vi "主界面.vi"() -> ()   [LabVIEW 2018]
panel:
  in  "配置文件":path=path "D:/Labviewprogram/多账户登录"
  in  "修改密码":bool
  in  "进入系统":bool
  in  "用户管理":bool
  in  "退出":bool
  in  "登录":bool
  in  "密 码":string
  in  "账 户":u16(ring)
  # "登录系统"
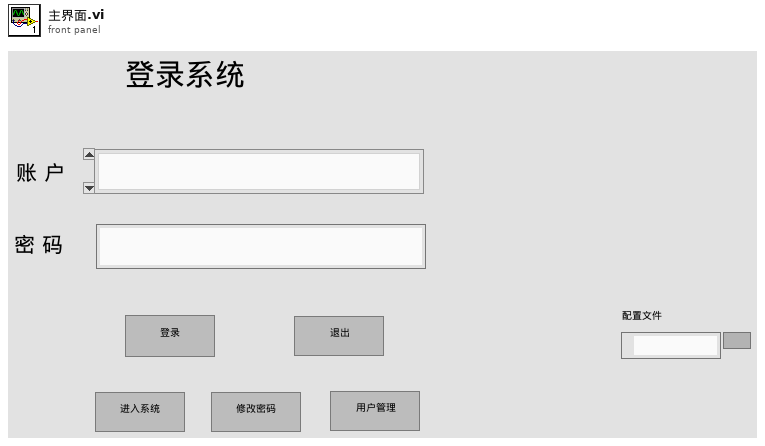
[diagram p1: front panel]
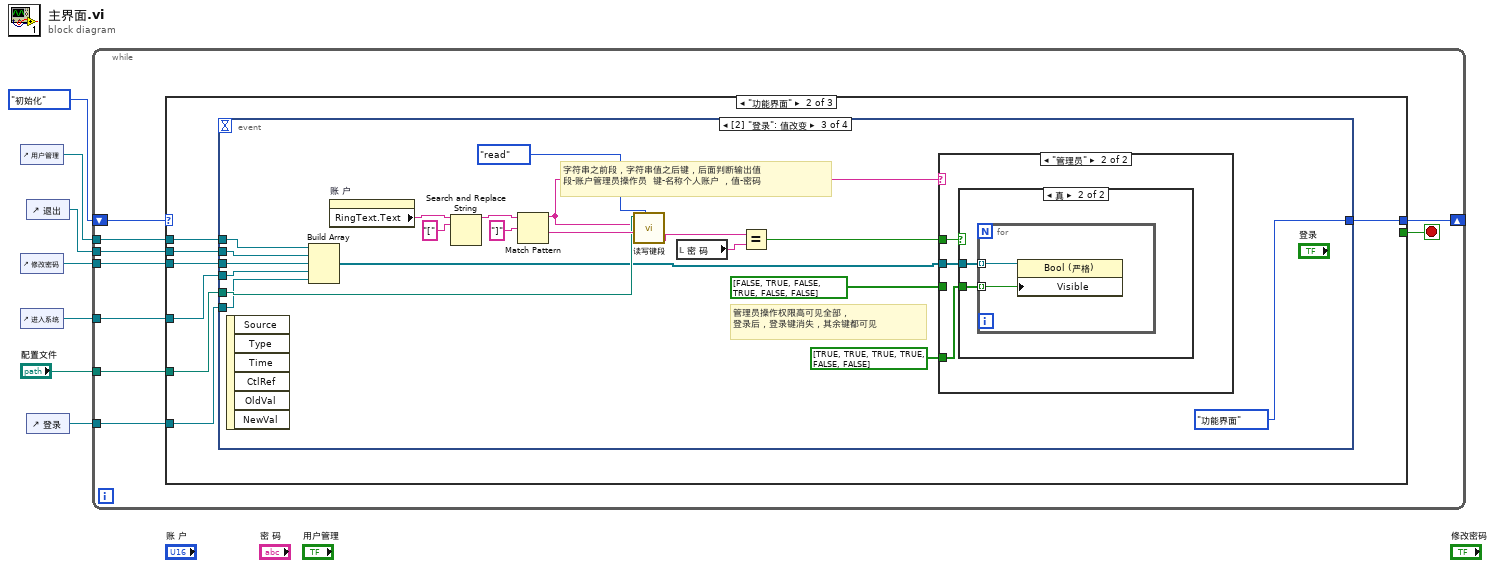
[diagram p0: block diagram]
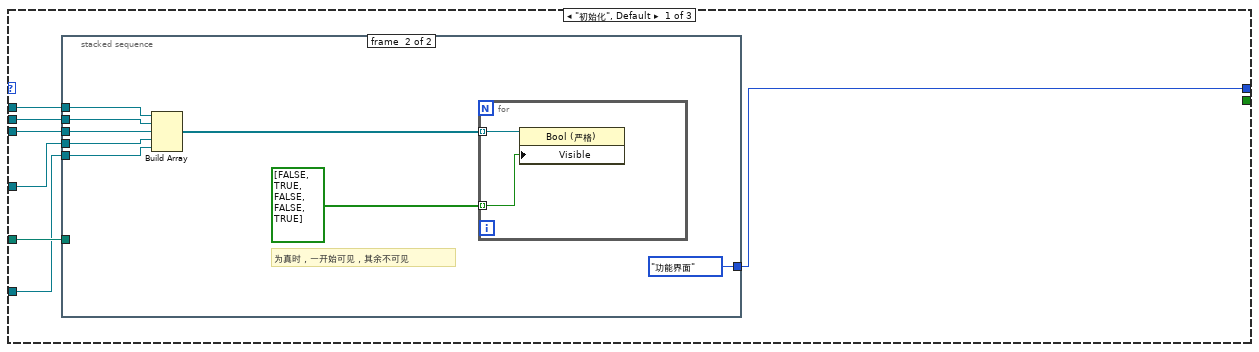
[diagram p2: hidden frame]
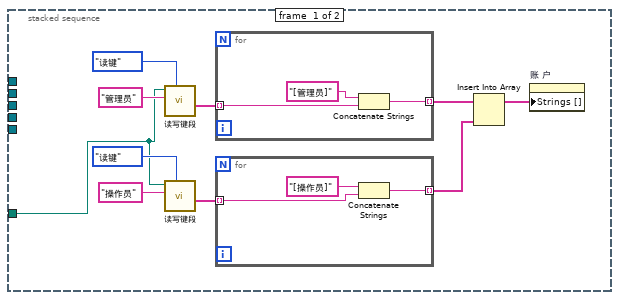
[diagram p3: hidden frame]
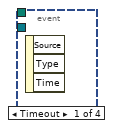
[diagram p4: hidden frame]
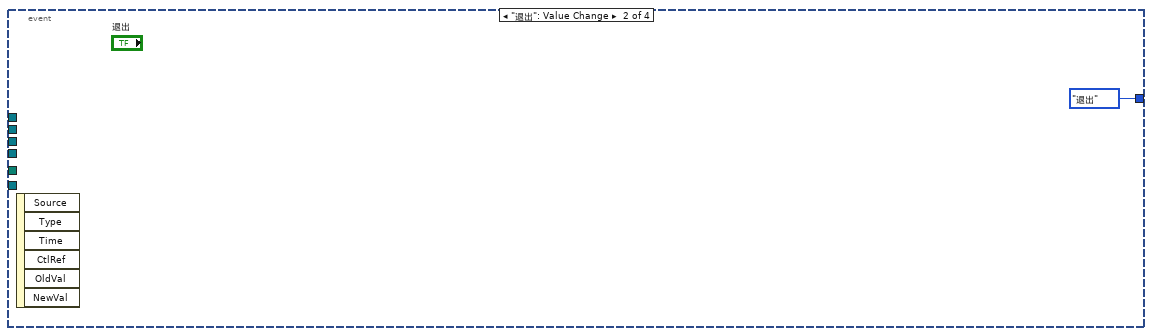
[diagram p5: hidden frame]
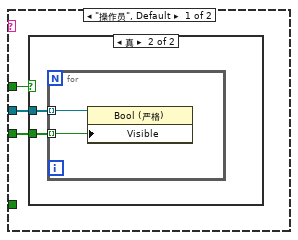
[diagram p6: hidden frame]
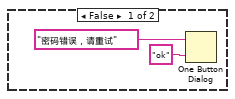
[diagram p7: hidden frame]
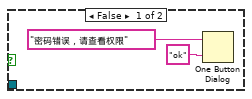
[diagram p8: hidden frame]
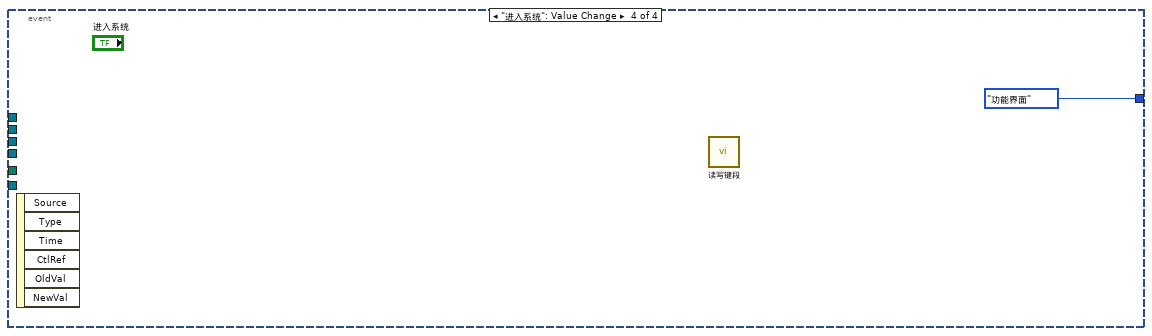
[diagram p9: hidden frame]
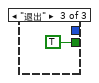
[diagram p10: hidden frame]
diagram:
  n1 = control-ref of="用户管理"() -> (w5:refnum<vi>)
  n2 = control-ref of="修改密码"() -> (w3:refnum<vi>)
  n3 = control-ref of="进入系统"() -> (w2:refnum<vi>)
  n4 = control-ref of="退出"() -> (w4:refnum<vi>)
  n5 = control-ref of="登录"() -> (w1:refnum<vi>)
  n6 = while {
    shift-right: [w9] -> _
    shift-left: enum16{"初始化", "功能界面", "退出"}."初始化" ("枚举") -> [w16]
    tunnel: "配置文件" -> [w15]
    tunnel: w5 -> [w14]
    tunnel: w4 -> [w13]
    tunnel: w3 -> [w12]
    tunnel: w2 -> [w11]
    tunnel: w1 -> [w10]
    stop <- w8 stop-if-true
    n7 = case shown="\"功能界面\"" w16 {
      tunnel: w15 -> [w23 w55 _]
      tunnel: w14 -> [w22 w54 _]
      tunnel: w13 -> [w21 w53 _]
      tunnel: w12 -> [w20 w52 _]
      tunnel: w11 -> [w19 w51 _]
      tunnel: w10 -> [w18 w50 _]
      tunnel: [w17 w56 _] -> w9
      tunnel: [_ _ TRUE] -> w8
      frame "初始化", Default {
        n8 = stacked-sequence {
          tunnel: w23 -> [w27 _]
          tunnel: w22 -> [_ w47]
          tunnel: w21 -> [_ w46]
          tunnel: w20 -> [_ w45]
          tunnel: w19 -> [_ w44]
          tunnel: w18 -> [_ w43]
          tunnel: [_ enum16{"初始化", "功能界面", "退出"}."功能界面" ("枚举")] -> w17
          frame #0 {
            n9 = call "读写键段.vi"("枚举"=enum16{"write", "read", "读键", "读段"}."读键", "段"="管理员", "配置文件"=w27) -> ("键名"=w31:string[])  [unwired: 6 in, 2 out]
            n10 = call "读写键段.vi"("枚举"=enum16{"write", "read", "读键", "读段"}."读键", "段"="操作员", "配置文件"=w27) -> ("键名"=w30:string[])  [unwired: 6 in, 2 out]
            n11 = for {
              tunnel: w31 -> [w38] mode=indexing
              tunnel: [w37] -> w26 mode=indexing
              n12 = Concatenate Strings("[管理员]" ("字符串"), w38) -> (w37:string)
            }
            n13 = for {
              tunnel: w30 -> [w35] mode=indexing
              tunnel: [w34] -> w25 mode=indexing
              n14 = Concatenate Strings("[操作员]" ("字符串"), w35) -> (w34:string)
            }
            n15 = Insert Into Array(array=w26, new element=w25) -> (w24:string[])  [unwired: 1 in]
            n16 = property on="账 户" class="Ring (严格)"("Strings []"=w24) -> ()  [unwired: 2 in, 2 out]
          }
          frame #1 {
            # "为真时，一开始可见，其余不可见"
            n17 = Build Array(w47, w46, w45, w44, w43) -> (w42:refnum<vi>[])
            n18 = for {
              tunnel: w42 -> [w49] mode=indexing
              tunnel: bool[] [FALSE, TRUE, FALSE, FALSE, TRUE] -> [w48] mode=indexing
              n19 = property class="Bool (严格)"(reference=w49, "Visible"=w48) -> ()  [unwired: 1 in, 2 out]
            }
          }
        }
      }
      frame "功能界面" {
        n20 = event shown="[2] \"登录\": 值改变" {
          selector: _ -> [_ _ _ _]
          dyn-events: _ -> [_ _ _ _]
          timeout: _ -> [_ _ _ _]
          tunnel: [_ enum16{"初始化", "功能界面", "退出"}."退出" ("枚举") enum16{"初始化", "功能界面", "退出"}."功能界面" ("枚举") enum16{"初始化", "功能界面", "退出"}."功能界面" ("枚举")] -> w56
          tunnel: w55 -> [_ _ w71 _]
          tunnel: w54 -> [_ _ w66 _]
          tunnel: w53 -> [_ _ w65 _]
          tunnel: w52 -> [_ _ w64 _]
          tunnel: w51 -> [_ _ w63 _]
          tunnel: w50 -> [_ _ w62 _]
          event Timeout {
            n21 = event-data() -> ()  [unwired: 1 in, 3 out]
          }
          event "退出": Value Change {
            n22 = event-data() -> ()  [unwired: 1 in, 6 out]
          }
          event "登录": Value Change {
            # "管理员操作权限高可见全部，\n登录后，登录键消失，其余键都可见"
            # "字符串之前段，字符串值之后键，后面判断输出值\n段-账户管理员操作员  键-名称个人账户 ，值-密码"
            n23 = event-data() -> ()  [unwired: 1 in, 6 out]
            n24 = Build Array(w66, w65, w64, w63, w62) -> (w61:refnum<vi>[])
            n25 = property on="账 户" class="Ring (严格)"() -> ("RingText.Text"=w77:string)  [unwired: 2 in, 2 out]
            n26 = Search and Replace String(input string=w77, search string="[" ("搜索字符串")) -> (result string=w75:string)  [unwired: 6 in, 3 out]
            n27 = Match Pattern(string=w75, regular expression="]" ("正则表达式")) -> (before substring=w69:string, after substring=w73:string)  [unwired: 1 in, 2 out]
            n28 = call "读写键段.vi"("枚举"=enum16{"write", "read", "读键", "读段"}."read", "key"=w73, "段"=w69, "配置文件"=w71) -> ("读取值"=w67:string)  [unwired: 5 in, 2 out]
            n29 = local read "密 码"() -> (w70:string)
            n30 = Equal?(x=w67, y=w70) -> (x = y?=w68:bool)
            n31 = case shown="\"管理员\"" w69 {
              tunnel: w68 -> [w80 w89]
              tunnel: w61 -> [w79 w88]
              tunnel: bool[] [TRUE, TRUE, TRUE, TRUE, FALSE, FALSE] -> [_ w87]
              tunnel: bool[] [FALSE, TRUE, FALSE, TRUE, FALSE, FALSE] -> [w78 _]
              frame "操作员", Default {
                n32 = case shown="真" w80 {
                  tunnel: w79 -> [_ w84]
                  tunnel: w78 -> [_ w83]
                  frame False {
                    n33 = One Button Dialog(message="密码错误，请重试" ("消息"), button name ("OK")="ok" ("按钮名称（“确定”）")) -> ()  [unwired: 1 out]
                  }
                  frame True {
                    n34 = for {
                      tunnel: w84 -> [w86] mode=indexing
                      tunnel: w83 -> [w85] mode=indexing
                      n35 = property class="Bool (严格)"(reference=w86, "Visible"=w85) -> ()  [unwired: 1 in, 2 out]
                    }
                  }
                }
              }
              frame "管理员" {
                n36 = case shown="真" w89 {
                  tunnel: w88 -> [_ w93]
                  tunnel: w87 -> [_ w92]
                  frame False {
                    n37 = One Button Dialog(message="密码错误，请查看权限" ("消息"), button name ("OK")="ok" ("按钮名称（“确定”）")) -> ()  [unwired: 1 out]
                  }
                  frame True {
                    n38 = for {
                      tunnel: w93 -> [w95] mode=indexing
                      tunnel: w92 -> [w94] mode=indexing
                      n39 = property class="Bool (严格)"(reference=w95, "Visible"=w94) -> ()  [unwired: 1 in, 2 out]
                    }
                  }
                }
              }
            }
          }
          event "进入系统": Value Change {
            n40 = event-data() -> ()  [unwired: 1 in, 6 out]
            n41 = call "读写键段.vi"() -> ()  [unwired: 9 in, 3 out]
          }
        }
      }
      frame "退出" {
      }
    }
  }
